vi "Set Start Trigger.vi"   [LabVIEW 2020, in "NI_VS Data Logging API.lvlib"]
doc: "Specifies a trigger condition on which to start logging data. You also can specify whether to log channel data immediately preceding the trigger condition and whether logging is retriggerable, meaning the data logging session watches for subsequent occurrences of the start trigger after the first logging operation finishes. By default, logging stops after one operation.\n\nYou must manually select the polymorphic instance to use."
uses:
  <vilib>/NI VeriStand/Execution/DataLogging/NI_VS Data Logging API.lvlib
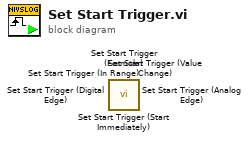
[diagram p0: block diagram]
diagram:
  n1 = call <vilib>:"Set Start Trigger (Start Immediately).vi"() -> ()  [unwired: 10 in, 2 out]
  n2 = call <vilib>:"Set Start Trigger (Value Change).vi"() -> ()  [unwired: 10 in, 2 out]
  n3 = call <vilib>:"Set Start Trigger (Digital Edge).vi"() -> ()  [unwired: 10 in, 2 out]
  n4 = call <vilib>:"Set Start Trigger (Analog Edge).vi"() -> ()  [unwired: 10 in, 2 out]
  n5 = call <vilib>:"Set Start Trigger (In Range).vi"() -> ()  [unwired: 10 in, 2 out]
  n6 = call <vilib>:"Set Start Trigger (Formula).vi"() -> ()  [unwired: 10 in, 2 out]
